vi "send&receive_BigRndArr.vi"() -> ()   [LabVIEW 2018, in "LabView-0mq-Jl_Roundtrip_lib.lvlib"]
uses:
  LabView-0mq-Jl_Roundtrip_lib.lvlib
  Server or client state.ctl
  detailed error info.ctl
  StackFrame.ctl
  Commands v2.ctl
  commands LV2Jl.ctl
  0a40c323-4a6a-4cac-b0a4-3ac9ee9fea3a.vi
  d2cb43a9-9305-42fb-ad58-bce983510195.vi
  c408c7c2-657c-47b6-beae-5b528cf4b72f.vi
  0a40c323-4a6a-4cac-b0a4-3ac9ee9fea3a.vi/cff2d2b7-9160-4f4a-b735-5eb6f847a7f3.vi
  d2cb43a9-9305-42fb-ad58-bce983510195.vi/cf934324-c94f-44b4-90db-ed3279dce7e0.vi
  d2cb43a9-9305-42fb-ad58-bce983510195.vi/e8094900-a7e5-4deb-a661-9091dfdad77c.vi
  d2cb43a9-9305-42fb-ad58-bce983510195.vi/cce96510-ab96-46c5-8576-6bbba9dc6d4d.vi
  c408c7c2-657c-47b6-beae-5b528cf4b72f.vi/77135d94-6f96-4a78-a1fc-58f76e985a97.vi
  c408c7c2-657c-47b6-beae-5b528cf4b72f.vi/6a593baf-46df-43dc-ba4a-8a2950bdaa8b.vi
  0a40c323-4a6a-4cac-b0a4-3ac9ee9fea3a.vi/cff2d2b7-9160-4f4a-b735-5eb6f847a7f3.vi/4d1245e0-8c93-46a3-96b0-1454c80dee4a.vi
  c408c7c2-657c-47b6-beae-5b528cf4b72f.vi/77135d94-6f96-4a78-a1fc-58f76e985a97.vi/9e6b7bb6-a7f0-4a12-9ca8-7d9b72990ca5.vi
  c408c7c2-657c-47b6-beae-5b528cf4b72f.vi/77135d94-6f96-4a78-a1fc-58f76e985a97.vi/cfe17dee-421c-42b6-a421-581ab5033fb8.vi
  0a40c323-4a6a-4cac-b0a4-3ac9ee9fea3a.vi/cff2d2b7-9160-4f4a-b735-5eb6f847a7f3.vi/4d1245e0-8c93-46a3-96b0-1454c80dee4a.vi/8a491148-96bd-425e-bebb-d3374d3dfcab.vi
  c408c7c2-657c-47b6-beae-5b528cf4b72f.vi/77135d94-6f96-4a78-a1fc-58f76e985a97.vi/9e6b7bb6-a7f0-4a12-9ca8-7d9b72990ca5.vi/be3a7147-190f-4342-b2ba-0d8d91cd1472.vi
  check ID validity.vi
  bindata_descr to JSON.vi
  check cluster field names.vi
  concat JSON.vi
  <vilib>/Utility/error.llb/Error Cluster From Error Code.vi
panel:
  out "roundtrip, ms/MB":dbl
  out "time to build req":dbl
  out "time, parse resp":dbl
  out "data size (Byte)":i32 format="%.0p"
  out "time roundtrip":dbl
  in  "dim 2":i32=100
  in  "dim 1":i32=100
  in  "showversion":bool=TRUE
  out "detailed error info":T1
  out "arr element":cdb
  out "numarray 2D":dbl[][](array[numeric])
  in  "index to return":cluster{"idx":u16[]}={"idx"=[1, 1, 1]} {"idx" min=1}
  in  "stop LV only":bool
  out "Jl Server state out":T3
  out "short err code":u8
  in  "go once":bool
  out "final error":errorcluster
  out "current error":errorcluster
  in  "stop":bool
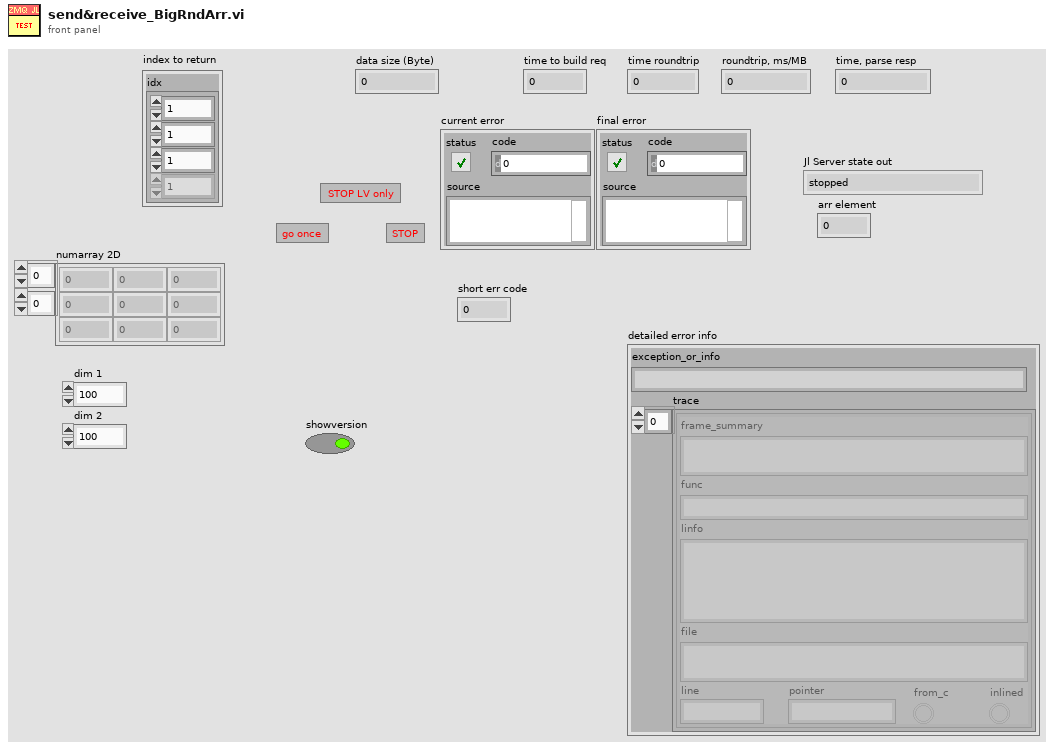
[diagram p1: front panel]
types:
  T1 = typedef "LabView-0mq-Jl_Roundtrip_lib.lvlib/detailed error info.ctl" = cluster{"exception_or_info":string, "trace":T2[]}
  T2 = typedef "LabView-0mq-Jl_Roundtrip_lib.lvlib/StackFrame.ctl" = cluster{"frame_summary":string, "func":string, "linfo":string, "file":string, "line":i32, "pointer":u64, "from_c":bool, "inlined":bool}
  T3 = typedef "LabView-0mq-Jl_Roundtrip_lib.lvlib/Server or client state.ctl" = enum16{"stopped", "running", "unknown"}
  T4 = typedef "LabView-0mq-Jl_Roundtrip_lib.lvlib/Commands v2.ctl" = enum16{"Start Jl-server & Init LV-client", "Send request & Get response ", "Stop Jl-server & Cleanup LV-client", "Cleanup LV-client", "Start Jl-server", "Stop Jl-server", "Init LV-Client", "Cleanup LV-Client", "(not allowed)", "Set LV Client state", "Set Jl Server state"}
  T5 = typedef "commands LV2Jl.ctl" = u8
  T6 = typedef "Bindata&description.ctl" = cluster{"bindata_descr":T7[], "bindata":u8[]}
  T7 = typedef "LabView-0mq-Jl_Roundtrip_lib.lvlib/Bindata description.ctl" = cluster{"nofbytes":i32, "numtype":string, "start":i32, "arrdims":i32[], "kwarg_name":string, "category":string}
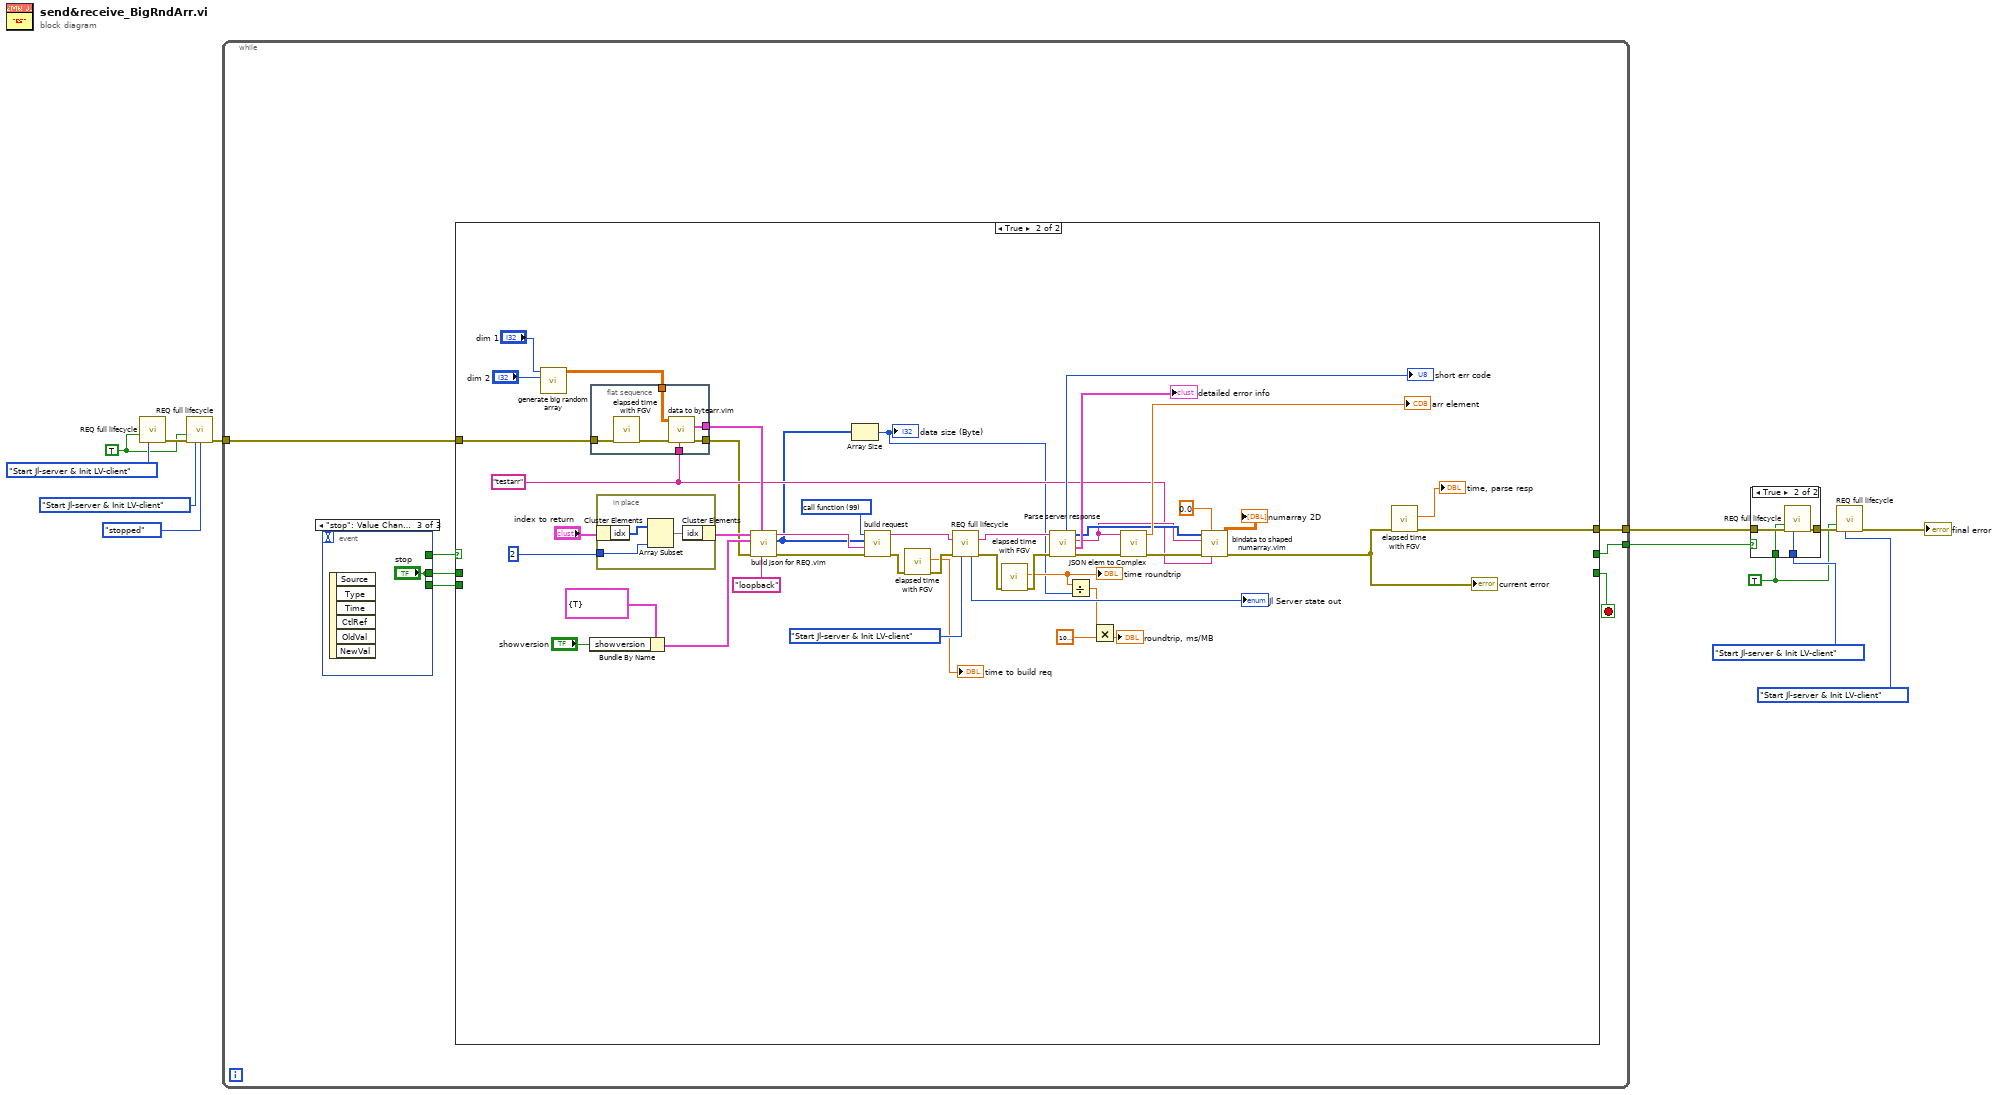
[diagram p0: block diagram]
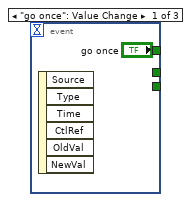
[diagram p3: hidden frame]
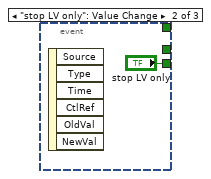
[diagram p4: hidden frame]
diagram:
  w2 = TRUE ("Force command")
  w8 = TRUE ("Force command")
  n1 = call "REQ full lifecycle.vi"("Force command"=w2, "command"=Commands_v2."Start Jl-server & Init LV-client") -> ("error out"=w4:errorcluster)  [unwired: 10 in, 3 out]
  n2 = call "REQ full lifecycle.vi"("Force command"=w2, "error in"=w4, "command"=Commands_v2."Start Jl-server & Init LV-client", "Jl Server state in"=Server_or_client_state."stopped") -> ("error out"=w6:errorcluster)  [unwired: 8 in, 3 out]
  n3 = while {
    tunnel: w6 -> [w14]
    tunnel: [w18] -> w13
    tunnel: [w19] -> w7
    stop <- w20 stop-if-true
    n4 = event shown="[2] \"stop\": Value Change" {
      selector: _ -> [_ _ _]
      dyn-events: _ -> [_ _ _]
      timeout: _ -> [_ _ _]
      tunnel: [_ "stop LV only" "stop"] -> w16
      tunnel: [_ _ "stop"] -> w15
      tunnel: ["go once" _ _] -> w17
      event "go once": Value Change {
        n5 = event-data() -> ()  [unwired: 1 in, 6 out]
      }
      event "stop LV only": Value Change {
        n6 = event-data() -> ()  [unwired: 1 in, 6 out]
      }
      event "stop": Value Change {
        n7 = event-data() -> ()  [unwired: 1 in, 6 out]
      }
    }
    n8 = case shown="True" w17 {
      tunnel: [w26 _] -> w20
      tunnel: [w25 _] -> w19
      tunnel: [w24 w41] -> w18
      tunnel: w16 -> [w26 _]
      tunnel: w15 -> [w25 _]
      tunnel: w14 -> [w24 w40]
      frame False {
      }
      frame True {
        w44 = "testarr" ("Tag")
        w67 = T5 99 items=["call function"=99, "ping"=112, "stop"=115] ("Command")
        n9 = call "generate big random array.vi"("dim 2"="dim 2", "dim 1"="dim 1") -> ("Array"=w51:dbl[][])  [unwired: 9 in]
        n10 = Bundle By Name(cluster=cluster{"showversion":bool} {"showversion"=TRUE}, "showversion"="showversion") -> (w53:cluster{"showversion":bool})
        n11 = flat-sequence {
          tunnel: [w76] -> w52
          tunnel: w51 -> [w75]
          tunnel: w44 -> [w74]
          tunnel: w40 -> [w71]
          tunnel: [w73] -> w33
          frame #0 {
            n12 = call "elapsed time with FGV.vi"("error in (no error)"=w71) -> ("error out"=w72:errorcluster)  [unwired: 9 in, 1 out]
            n13 = call "data to bytearr.vim"("kwarg_name"=w74, "error in (no error)"=w72, "data in"=w75) -> ("error out"=w73:errorcluster, "Bindata & descr out"=w76:T6)  [unwired: 6 in, 1 out]
          }
        }
        n14 = in-place {
          in-place-border: u8 2 ("dims") -> [w78]
          n15 = in-place-cluster #1("index to return") -> ("idx"=w79:u16[])
          n16 = Array Subset(array=w79, length=w78) -> (w77:u16[])  [unwired: 1 in]
          n17 = in-place-cluster #1("idx"=w77) -> (w61:cluster{"idx":u16[]})
        }
        n18 = call "build json for REQ.vim"("fun2call"="loopback", "Bindata & descr in"=w52, "error in (no error)"=w33, "Arguments 2"=w53, "Arguments 1"=w61) -> ("error out"=w70:errorcluster, "bindata out"=w39:u8[], "JSON string out"=w63:string)  [unwired: 4 in]
        n19 = Array Size(array=w39) -> (size(s)=w30:i32)
        "data size (Byte)" <- w30
        n20 = call "build request.vi"("error in (no error)"=w70, "JSON data"=w63, "binary data"=w39, "Command"=w67) -> ("error out"=w38:errorcluster, "REQ string"=w69:string)  [unwired: 6 in]
        n21 = call "elapsed time with FGV.vi"("error in (no error)"=w38) -> ("error out"=w37:errorcluster, "elapsed time, s"=→"time to build req":dbl)  [unwired: 9 in]
        n22 = call "REQ full lifecycle.vi"("data to send"=w69, "error in"=w37, "command"=Commands_v2."Start Jl-server & Init LV-client") -> ("server response"=w65:string, "Jl Server state out"=→"Jl Server state out":T3, "error out"=w36:errorcluster)  [unwired: 9 in, 1 out]
        n23 = call "elapsed time with FGV.vi"("error in (no error)"=w36) -> ("error out"=w35:errorcluster, "elapsed time, s"=w31:dbl)  [unwired: 9 in]
        "time roundtrip" <- w31
        n24 = call "Parse server response.vi"("error in (no error)"=w35, "server response in"=w65) -> ("error out"=w58:errorcluster, "detailed error info"=→"detailed error info":T1, "JSON out"=w46:string, "binary data"=w47:u8[], "return code"=→"short err code":u8)  [unwired: 3 in, 2 out]
        n25 = Divide(x=w31, y=w30) -> (x/y=w29:dbl)
        n26 = Multiply(x=w29, y=1000000000.0 ("x")) -> (x*y=→"roundtrip, ms/MB":dbl)
        n27 = call "JSON elem to Complex.vi"("error in (no error)"=w58, "JSON in"=w46) -> ("error out"=w48:errorcluster, "Numeric"=→"arr element":cdb)  [unwired: 8 in]
        n28 = call "bindata to shaped numarray.vim"("kwarg_name"=w44, "data type"=0.0, "error in (no error)"=w48, "bindata_descr"=w46, "binary data"=w47) -> ("error out"=w42:errorcluster, "numarray 2D"=→"numarray 2D":dbl[][])  [unwired: 3 in, 2 out]
        "current error" <- w42
        n29 = call "elapsed time with FGV.vi"("error in (no error)"=w42) -> ("error out"=w41:errorcluster, "elapsed time, s"=→"time, parse resp":dbl)  [unwired: 9 in]
      }
    }
  }
  n30 = case shown="True" w7 {
    tunnel: w13 -> [w80 w84]
    tunnel: Commands_v2."Start Jl-server & Init LV-client" ("command") -> [_ w83]
    tunnel: [w80 w82] -> w11
    tunnel: w8 -> [_ w81]
    frame False {
    }
    frame True {
      n31 = call "REQ full lifecycle.vi"("Force command"=w81, "error in"=w84, "command"=w83) -> ("error out"=w82:errorcluster)  [unwired: 9 in, 3 out]
    }
  }
  n32 = call "REQ full lifecycle.vi"("Force command"=w8, "error in"=w11, "command"=Commands_v2."Start Jl-server & Init LV-client") -> ("error out"=→"final error":errorcluster)  [unwired: 9 in, 3 out]
